vi "user32_MessageBoxA.vi"() -> ()   [LabVIEW 2013]
uses:
  User32.dll
panel:
  out "返回类型":i32
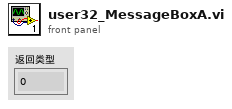
[diagram p1: front panel]
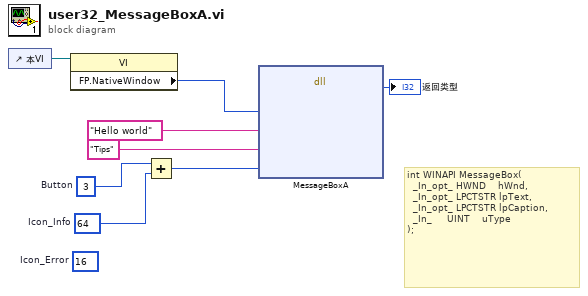
[diagram p0: block diagram]
diagram:
  (unwired) u8 16  # Icon_Error
  w2 = u8 64  # Icon_Info
  w6 = u8 3  # Button
  # "int WINAPI MessageBox(\n  _In_opt_ HWND    hWnd,\n  _In_opt_ LPCTSTR lpText,\n  _In_opt_ LPCTSTR lpCaption,\n  _In_     UINT    uType\n);"
  n1 = control-ref of="本VI"() -> (w4:refnum<vi>)
  n2 = property class="VI"(reference=w4) -> ("FP.NativeWindow"=w1:u64)  [unwired: 1 in, 2 out]
  n3 = Add(x=w6, y=w2) -> (x+y=w3:u8)
  n4 = dll-call lib="User32.dll" fn="MessageBoxA"("hWnd"=w1, "lpText"="Hello world", "Title"="Tips", "Type"=w3) -> ("返回类型"=→"返回类型":i32)  [unwired: 7 in, 2 out]
